vi "Get Gain Auto.vi"(8 "error in (no error)":errorcluster, 11 "Camera in":refnum<class "Camera.lvclass">) -> (0 "error out":errorcluster, 2 "Mode":T1, 3 "Camera":refnum<class "Camera.lvclass">)   [LabVIEW 2020, in "Camera.lvclass"]
uses:
  Camera.lvclass
  Auto Mode.ctl
  Camera.lvclass/Camera.ctl
  Check Not Disconnected.vi
  <vilib>/Utility/error.llb/Error Cluster From Error Code.vi
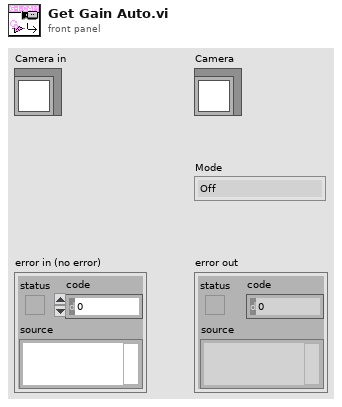
[diagram p1: front panel]
types:
  T1 = typedef "Camera.lvclass/Auto Mode.ctl" = enum8{"Off", "Once", "Continuous"}
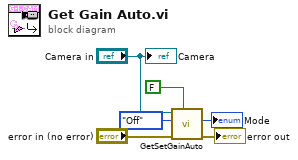
[diagram p0: block diagram]
diagram:
  n1 = call "GetSetGainAuto.vi"("Set?"=FALSE, "error in (no error)"="error in (no error)", "Auto Mode"=Auto_Mode."Off", "Camera in"="Camera in") -> ("error out"=→"error out":errorcluster, "Mode"=→"Mode":T1)  [unwired: 6 in]
  "Camera" <- "Camera in"
